vi "Sciteq GPIB driver.vi"(1 "?":cluster{sgl, sgl, sgl, sgl}={44.0, 0.20000002, 0.0, 0.0} {"?" min=0 max=0.009 step=0.001 scale=0.0..0.009 scale format="%.3f"; "?" min=0 max=0.09 step=0.01 scale=0.0..0.09 scale format="%.2f"; "?" min=0 max=0.9 step=0.1 scale=0.0..0.9 scale format="%.1f"; "?" min=0 max=320 step=1 scale=0.0..320.0}) -> (0 "frequency":sgl format="%.2f")   [LabVIEW 2022 SP3]
panel:
  in  "ON":bool=TRUE
  in  "?":dbl(knob)=45000000.0 min=1000000.0 max=320000000.0 step=10000.0 scale=1000000.0..320000000.0 scale format="%.2e"
  out "GPIB command":string="X04800000Y01"
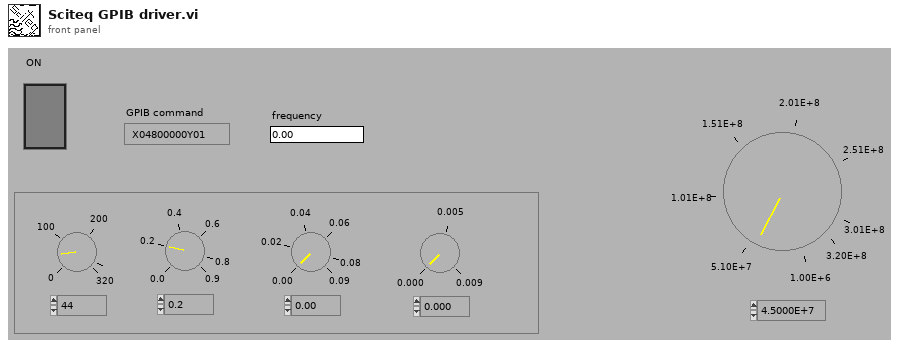
[diagram p1: front panel]
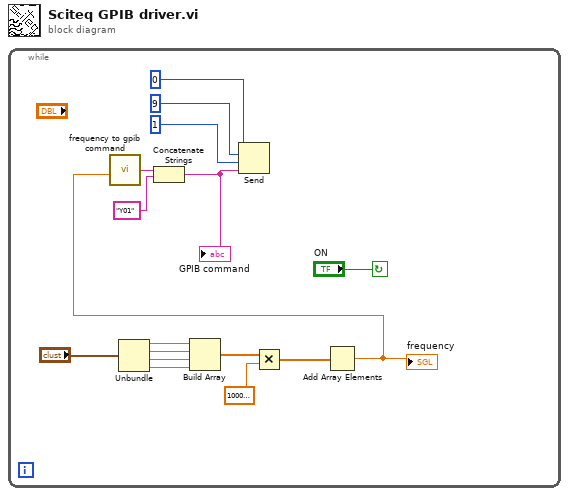
[diagram p0: block diagram]
diagram:
  n1 = while {
    stop <- "ON" continue-if-true
    n2 = Unbundle("?") -> (w3:sgl, w4:sgl, w5:sgl, w6:sgl)
    n3 = Build Array(w3, w4, w5, w6) -> (w7:sgl[])
    n4 = Multiply(x=w7, y=sgl 1000000.0) -> (x*y=w9:sgl[])
    n5 = Add Array Elements(numeric array=w9) -> (sum=w1:sgl)
    "frequency" <- w1
    n6 = call "frequency to gpib command.vi"("Input Frequency"=w1) -> ("Final GPIB Command"=w15:string)
    n7 = Concatenate Strings(w15, "Y01") -> (w12:string)
    "GPIB command" <- w12
    n8 = Send(0:0, 2:i16 9, 3:u8 1, 5:w12) -> ()  [unwired: 1 in, 3 out]
  }
